vi "CANOpen_SetGet PDO Parameter Settings.vi"(6 "Set Parameters":bool, 8 "error in (no error)":errorcluster, 10 "Parameters":variant, 11 "PDO Parameter Settings":T1={"Parameter Name"="", "Scale Factor"=0.0, "Scale Offset"=0.0, "Byte Offset"=0, "Bit Offset"=0, "Data Type"=enum."U8", "Byte Order"=enum."little-endian"} {"Bit Offset" max=8 step=1; "Byte Offset" max=8 step=1}) -> (0 "error out":errorcluster, 2 "Parameters":variant, 3 "PDO Parameter Settings out":T1={"Parameter Name"="", "Scale Factor"=1.0, "Scale Offset"=0.0, "Byte Offset"=0, "Bit Offset"=0, "Data Type"=enum."U8", "Byte Order"=enum."little-endian"} {"Bit Offset" max=8 step=1; "Byte Offset" max=8 step=1})   [LabVIEW 2013, in "CANOpen Addon Custom Device.lvlib"]
uses:
  CANOpen Addon Custom Device.lvlib
  CANOpen_PDO Parameter Settings.ctl
  CANOpen_PDO Data Type.ctl
  System Explorer/SubVIs/CANopen Byte Order.ctl
  CANOpen Addon GUID Lookup Global.vi
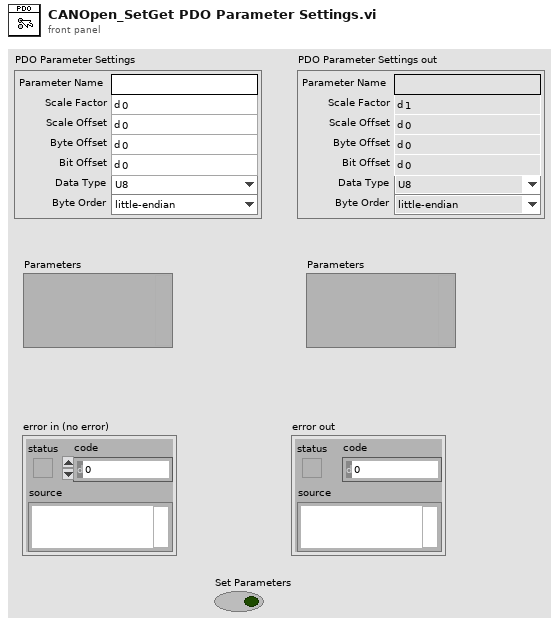
[diagram p1: front panel]
types:
  T1 = typedef "CANOpen Addon Custom Device.lvlib/CANOpen_PDO Parameter Settings.ctl" = cluster{"Parameter Name":string, "Scale Factor":dbl, "Scale Offset":dbl, "Byte Offset":u8, "Bit Offset":u8, "Data Type":T2, "Byte Order":T3}
  T2 = typedef "CANOpen Addon Custom Device.lvlib/CANOpen_PDO Data Type.ctl" = enum16{"U8", "U16", "U32", "I8", "I16", "I32", "Single", "Double", "Boolean"}
  T3 = typedef "CANOpen Addon Custom Device.lvlib/CANopen Byte Order.ctl" = enum16{"big-endian network order", "little-endian"}
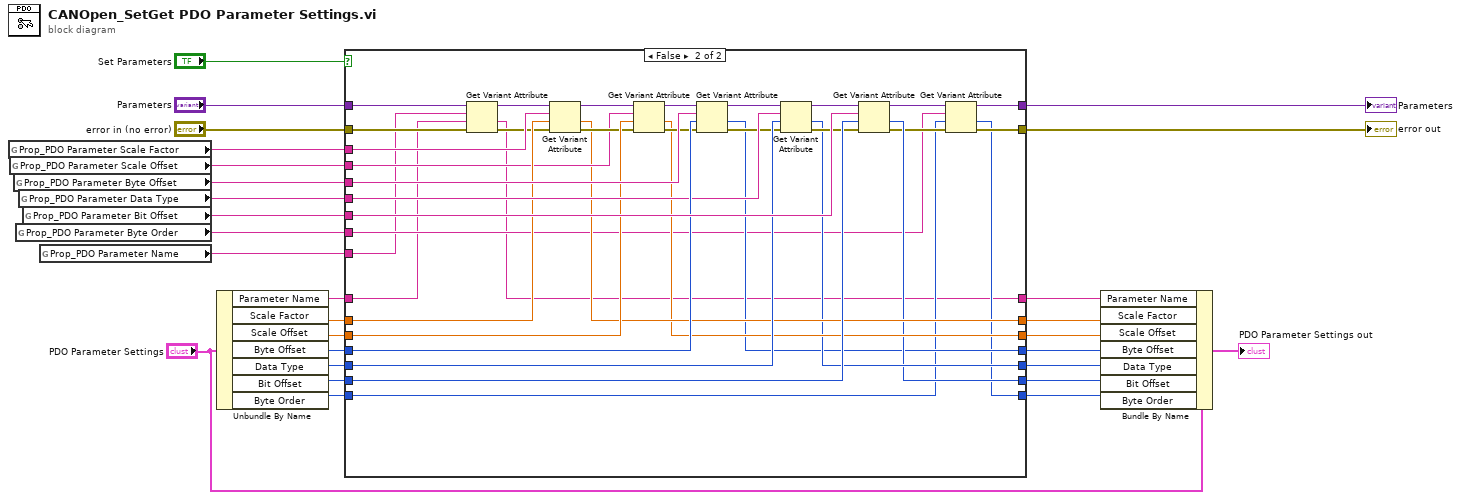
[diagram p0: block diagram]
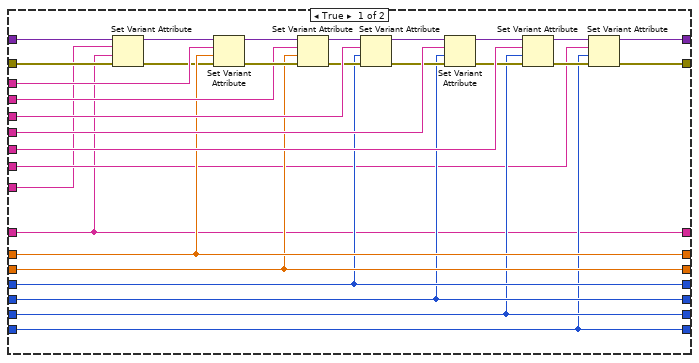
[diagram p2: hidden frame]
diagram:
  n1 = global read "CANOpen Addon GUID Lookup Global.vi" "Prop_PDO Parameter Scale Factor"() -> (w16:string)
  n2 = global read "CANOpen Addon GUID Lookup Global.vi" "Prop_PDO Parameter Scale Offset"() -> (w17:string)
  n3 = global read "CANOpen Addon GUID Lookup Global.vi" "Prop_PDO Parameter Byte Offset"() -> (w21:string)
  n4 = global read "CANOpen Addon GUID Lookup Global.vi" "Prop_PDO Parameter Byte Order"() -> (w4:string)
  n5 = global read "CANOpen Addon GUID Lookup Global.vi" "Prop_PDO Parameter Data Type"() -> (w22:string)
  n6 = global read "CANOpen Addon GUID Lookup Global.vi" "Prop_PDO Parameter Bit Offset"() -> (w28:string)
  n7 = global read "CANOpen Addon GUID Lookup Global.vi" "Prop_PDO Parameter Name"() -> (w1:string)
  n8 = Unbundle By Name("PDO Parameter Settings") -> ("Parameter Name"=w3:string, "Scale Factor"=w19:dbl, "Scale Offset"=w20:dbl, "Byte Offset"=w23:u8, "Data Type"=w24:T2, "Bit Offset"=w27:u8, "Byte Order"=w6:T3)
  n9 = case shown="False" "Set Parameters" {
    tunnel: w28 -> [w58 w95]
    tunnel: w27 -> [w41 w94]
    tunnel: [w37 w69] -> w26
    tunnel: [w39 w71] -> w25
    tunnel: w24 -> [w42 w91]
    tunnel: w23 -> [w43 w90]
    tunnel: w22 -> [w55 w89]
    tunnel: w21 -> [w54 w88]
    tunnel: w20 -> [w44 w83]
    tunnel: w19 -> [w45 w82]
    tunnel: "error in (no error)" -> [w31 w63]
    tunnel: w17 -> [w48 w80]
    tunnel: w16 -> [w46 w78]
    tunnel: "Parameters" -> [w32 w64]
    tunnel: [w45 w77] -> w12
    tunnel: [w44 w76] -> w11
    tunnel: [w42 w75] -> w9
    tunnel: [w41 w74] -> w8
    tunnel: [w43 w73] -> w10
    tunnel: w6 -> [w36 w67]
    tunnel: [w36 w66] -> w5
    tunnel: w4 -> [w35 w68]
    tunnel: w3 -> [w30 w61]
    tunnel: [w30 w60] -> w2
    tunnel: w1 -> [w29 w59]
    frame True {
      n10 = Set Variant Attribute(Variant=w32, name=w29, value=w30, error in=w31) -> (Variant out=w34:variant, error out=w33:errorcluster)  [unwired: 1 out]
      n11 = Set Variant Attribute(Variant=w34, name=w46, value=w45, error in=w33) -> (Variant out=w47:variant, error out=w49:errorcluster)  [unwired: 1 out]
      n12 = Set Variant Attribute(Variant=w47, name=w48, value=w44, error in=w49) -> (Variant out=w52:variant, error out=w53:errorcluster)  [unwired: 1 out]
      n13 = Set Variant Attribute(Variant=w52, name=w54, value=w43, error in=w53) -> (Variant out=w51:variant, error out=w50:errorcluster)  [unwired: 1 out]
      n14 = Set Variant Attribute(Variant=w51, name=w55, value=w42, error in=w50) -> (Variant out=w57:variant, error out=w56:errorcluster)  [unwired: 1 out]
      n15 = Set Variant Attribute(Variant=w57, name=w58, value=w41, error in=w56) -> (Variant out=w38:variant, error out=w40:errorcluster)  [unwired: 1 out]
      n16 = Set Variant Attribute(Variant=w38, name=w35, value=w36, error in=w40) -> (Variant out=w37:variant, error out=w39:errorcluster)  [unwired: 1 out]
    }
    frame False {
      n17 = Get Variant Attribute(Variant=w64, name=w59, default value (empty Variant)=w61, error in=w63) -> (duplicate Variant=w65:variant, value=w60:string, error out=w62:errorcluster)  [unwired: 1 out]
      n18 = Get Variant Attribute(Variant=w65, name=w78, default value (empty Variant)=w82, error in=w62) -> (duplicate Variant=w79:variant, value=w77:dbl, error out=w81:errorcluster)  [unwired: 1 out]
      n19 = Get Variant Attribute(Variant=w79, name=w80, default value (empty Variant)=w83, error in=w81) -> (duplicate Variant=w86:variant, value=w76:dbl, error out=w87:errorcluster)  [unwired: 1 out]
      n20 = Get Variant Attribute(Variant=w86, name=w88, default value (empty Variant)=w90, error in=w87) -> (duplicate Variant=w85:variant, value=w73:u8, error out=w84:errorcluster)  [unwired: 1 out]
      n21 = Get Variant Attribute(Variant=w85, name=w89, default value (empty Variant)=w91, error in=w84) -> (duplicate Variant=w93:variant, value=w75:T2, error out=w92:errorcluster)  [unwired: 1 out]
      n22 = Get Variant Attribute(Variant=w93, name=w95, default value (empty Variant)=w94, error in=w92) -> (duplicate Variant=w70:variant, value=w74:u8, error out=w72:errorcluster)  [unwired: 1 out]
      n23 = Get Variant Attribute(Variant=w70, name=w68, default value (empty Variant)=w67, error in=w72) -> (duplicate Variant=w69:variant, value=w66:T3, error out=w71:errorcluster)  [unwired: 1 out]
    }
  }
  "Parameters" <- w26
  "error out" <- w25
  n24 = Bundle By Name(cluster="PDO Parameter Settings", "Parameter Name"=w2, "Scale Factor"=w12, "Scale Offset"=w11, "Byte Offset"=w10, "Data Type"=w9, "Bit Offset"=w8, "Byte Order"=w5) -> (→"PDO Parameter Settings out":T1)
